vi "Teleop.vi"(10 "Match Info":T1={"Autonomous Elapsed Seconds"=0.0, "TeleOp Elapsed Seconds"=0.0, "Disabled Elapsed Seconds"=0.0, "Visited Autonomous"=FALSE, "Visited TeleOp"=FALSE, "Visited Disabled"=FALSE, "Autonomous Settings"={"Autonomous Style"=enum."Independent", "VI Refnum"=refnum}}, 11 "Call Context":T2) -> ()   [LabVIEW 2013]
doc: "This VI is called for each TeleOp packet received from the DS where the robot is not disabled. It is often used to read from the joysticks and update I/O or to update setpoints for timed control loops. It should complete and return within 20 milliseconds or it may miss DS packets."
uses:
  <vilib>/Rock Robotics/WPI/DriverStation/WPI_DriverStationDerivedRobotMode.ctl
  <vilib>/Rock Robotics/WPI/DriverStation/WPI_DriverStationMatch Info.ctl
  Robot Global Data.vi
  <vilib>/Rock Robotics/WPI/Joystick/WPI_JoystickGetSetRefNum.vi
panel:
  out "Button 12 Joy 4":bool
  out "Button 11 Joy 4":bool
  out "Button 10 Joy 4":bool
  out "Button 9 Joy 4":bool
  out "Button 8 Joy 4":bool
  out "Button 7 Joy 4":bool
  out "Button 6 Joy 4":bool
  out "Button 5 Joy 4":bool
  out "Button 4 Joy 4":bool
  out "Button 3 Joy 4":bool
  out "Button 2 Joy 4":bool
  out "Button 1 Joy 4":bool
  out "axis 4 Joy 4":dbl
  out "axis 3 (throttle) Joy 4":dbl
  out "axis 2 (y) Joy 4":dbl
  out "axis 1 (x) Joy 4":dbl
  out "Button 12 Joy 3":bool
  out "Button 11 Joy 3":bool
  out "Button 10 Joy 3":bool
  out "Button 9 Joy 3":bool
  out "Button 8 Joy 3":bool
  out "Button 7 Joy 3":bool
  out "Button 6 Joy 3":bool
  out "Button 5 Joy 3":bool
  out "Button 4 Joy 3":bool
  out "Button 3 Joy 3":bool
  out "Button 2 Joy 3":bool
  out "Button 1 Joy 3":bool
  out "axis 4 Joy 3":dbl
  out "axis 3 (throttle) Joy 3":dbl
  out "axis 2 (y) Joy 3":dbl
  out "axis 1 (x) Joy 3":dbl
  out "Button 12 Joy 2":bool
  out "Button 11 Joy 2":bool
  out "Button 10 Joy 2":bool
  out "Button 9 Joy 2":bool
  out "Button 8 Joy 2":bool
  out "Button 7 Joy 2":bool
  out "Button 6 Joy 2":bool
  out "Button 5 Joy 2":bool
  out "Button 4 Joy 2":bool
  out "Button 3 Joy 2":bool
  out "Button 2 Joy 2":bool
  out "Button 1 Joy 2":bool
  out "axis 4 Joy 2":dbl
  out "axis 3 (throttle) Joy 2":dbl
  out "axis 2 (y) Joy 2":dbl
  out "axis 1 (x) Joy 2":dbl
  out "Button 12 Joy 1":bool
  out "Button 11 Joy 1":bool
  out "Button 10 Joy 1":bool
  out "Button 9 Joy 1":bool
  out "Button 8 Joy 1":bool
  out "Button 7 Joy 1":bool
  out "Button 6 Joy 1":bool
  out "Button 5 Joy 1":bool
  out "Button 4 Joy 1":bool
  out "Button 3 Joy 1":bool
  out "Button 2 Joy 1":bool
  out "Button 1 Joy 1":bool
  out "axis 4 Joy":dbl
  out "axis 3 (throttle) Joy 1":dbl
  out "axis 2 (y) Joy 1":dbl
  out "axis 1 (x) Joy 1":dbl
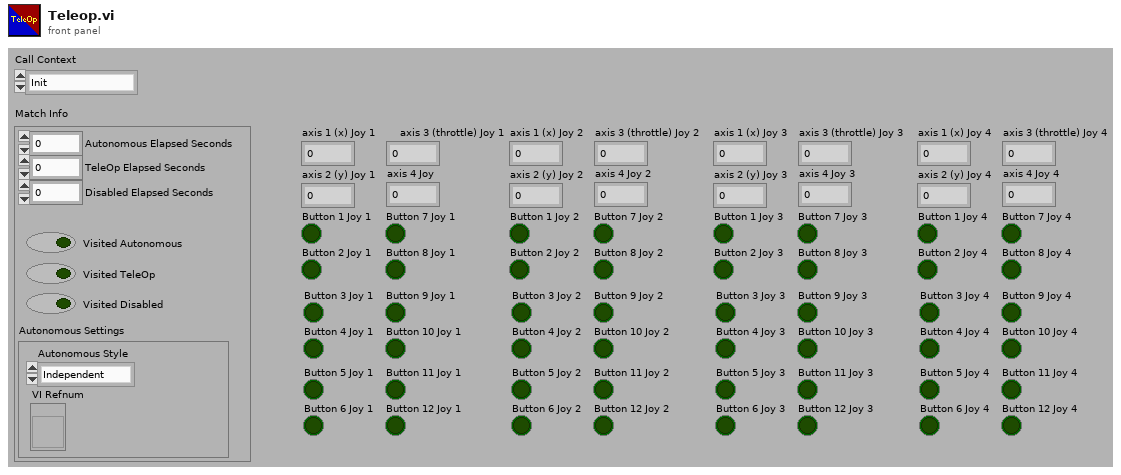
[diagram p1: front panel]
types:
  T1 = typedef "WPI_DriverStationMatch Info.ctl" = cluster{"Autonomous Elapsed Seconds":dbl, "TeleOp Elapsed Seconds":dbl, "Disabled Elapsed Seconds":dbl, "Visited Autonomous":bool, "Visited TeleOp":bool, "Visited Disabled":bool, "Autonomous Settings":cluster{"Autonomous Style":enum16{"Iterative", "Independent"}, "VI Refnum":refnum<vi>}}
  T2 = typedef "WPI_DriverStationDerivedRobotMode.ctl" = enum16{"Init", "Execute", "Stop"}
  T3 = typedef "WPI_JoystickDevRef.ctl" = cluster{"Device":T4}
  T4 = typedef "WPI_JoystickDeviceEnum.ctl" = enum16{"USB 1", "USB 2", "USB 3", "USB 4", "Kinect 1", "Kinect 2"}
  T5 = typedef "WPI_JoystickButtonState.ctl" = cluster{"Button 1":bool, "Button 2":bool, "Button 3":bool, "Button 4":bool, "Button 5":bool, "Button 6":bool, "Button 7":bool, "Button 8":bool, "Button 9":bool, "Button 10":bool, "Button 11":bool, "Button 12":bool}
  T6 = cluster{"axis 1 (x)":dbl, "axis 2 (y)":dbl, "axis 3 (throttle)":dbl, "axis 4":dbl, "axis 5":dbl, "axis 6":dbl}
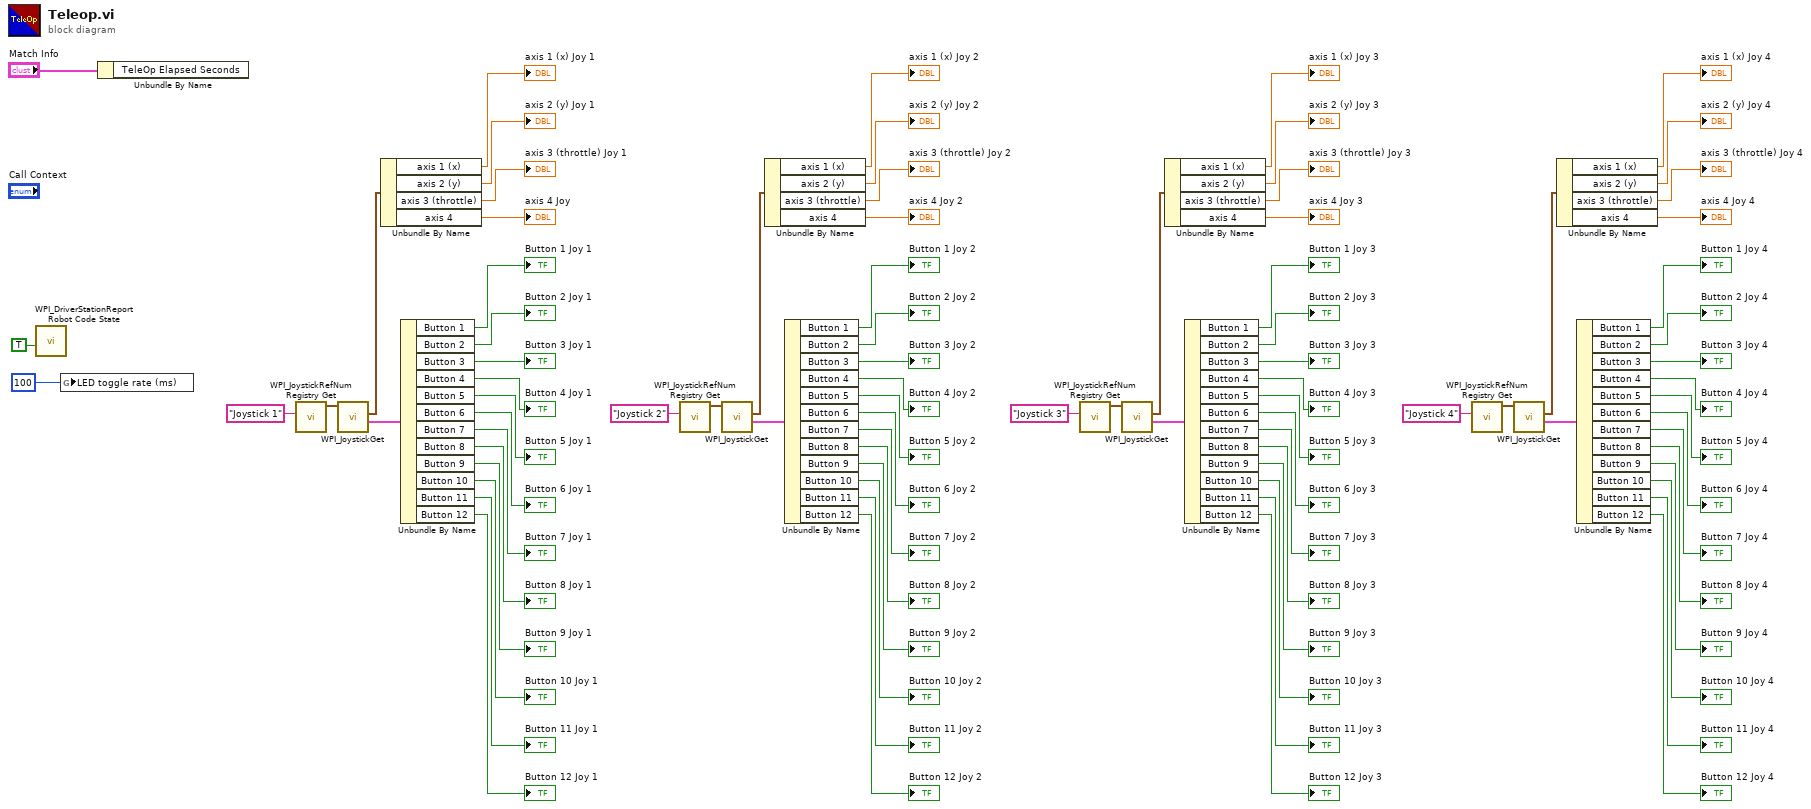
[diagram p0: block diagram]
diagram:
  n1 = call <vilib>:"WPI_DriverStationReport Robot Code State.vi"("TeleOp"=TRUE ("Autonomous")) -> ()  [unwired: 10 in, 1 out]
  n2 = global write "Robot Global Data.vi" "LED toggle rate (ms)"(u32 100 ("LED ms toggle rate")) -> ()
  n3 = Unbundle By Name("Match Info") -> ()  [unwired: 1 out]
  n4 = call <vilib>:"WPI_JoystickRefNum Registry Get.vi"("refnum name"="Joystick 1") -> ("JoystickDevRef"=w81:T3)  [unwired: 1 in, 9 out]
  n5 = call <vilib>:"WPI_JoystickGet.vi"("JoystickDevRef"=w81) -> ("Buttons"=w77:T5, "Axes"=w78:T6)  [unwired: 1 in, 4 out]
  n6 = Unbundle By Name(w78) -> ("axis 1 (x)"=→"axis 1 (x) Joy 1":dbl, "axis 2 (y)"=→"axis 2 (y) Joy 1":dbl, "axis 3 (throttle)"=→"axis 3 (throttle) Joy 1":dbl, "axis 4"=→"axis 4 Joy":dbl)
  n7 = Unbundle By Name(w77) -> ("Button 1"=→"Button 1 Joy 1":bool, "Button 2"=→"Button 2 Joy 1":bool, "Button 3"=→"Button 3 Joy 1":bool, "Button 4"=→"Button 4 Joy 1":bool, "Button 5"=→"Button 5 Joy 1":bool, "Button 6"=→"Button 6 Joy 1":bool, "Button 7"=→"Button 7 Joy 1":bool, "Button 8"=→"Button 8 Joy 1":bool, "Button 9"=→"Button 9 Joy 1":bool, "Button 10"=→"Button 10 Joy 1":bool, "Button 11"=→"Button 11 Joy 1":bool, "Button 12"=→"Button 12 Joy 1":bool)
  n8 = call <vilib>:"WPI_JoystickRefNum Registry Get.vi"("refnum name"="Joystick 2") -> ("JoystickDevRef"=w59:T3)  [unwired: 1 in, 9 out]
  n9 = call <vilib>:"WPI_JoystickGet.vi"("JoystickDevRef"=w59) -> ("Buttons"=w57:T5, "Axes"=w58:T6)  [unwired: 1 in, 4 out]
  n10 = Unbundle By Name(w58) -> ("axis 1 (x)"=→"axis 1 (x) Joy 2":dbl, "axis 2 (y)"=→"axis 2 (y) Joy 2":dbl, "axis 3 (throttle)"=→"axis 3 (throttle) Joy 2":dbl, "axis 4"=→"axis 4 Joy 2":dbl)
  n11 = Unbundle By Name(w57) -> ("Button 1"=→"Button 1 Joy 2":bool, "Button 2"=→"Button 2 Joy 2":bool, "Button 3"=→"Button 3 Joy 2":bool, "Button 4"=→"Button 4 Joy 2":bool, "Button 5"=→"Button 5 Joy 2":bool, "Button 6"=→"Button 6 Joy 2":bool, "Button 7"=→"Button 7 Joy 2":bool, "Button 8"=→"Button 8 Joy 2":bool, "Button 9"=→"Button 9 Joy 2":bool, "Button 10"=→"Button 10 Joy 2":bool, "Button 11"=→"Button 11 Joy 2":bool, "Button 12"=→"Button 12 Joy 2":bool)
  n12 = call <vilib>:"WPI_JoystickRefNum Registry Get.vi"("refnum name"="Joystick 3") -> ("JoystickDevRef"=w39:T3)  [unwired: 1 in, 9 out]
  n13 = call <vilib>:"WPI_JoystickGet.vi"("JoystickDevRef"=w39) -> ("Buttons"=w37:T5, "Axes"=w38:T6)  [unwired: 1 in, 4 out]
  n14 = Unbundle By Name(w38) -> ("axis 1 (x)"=→"axis 1 (x) Joy 3":dbl, "axis 2 (y)"=→"axis 2 (y) Joy 3":dbl, "axis 3 (throttle)"=→"axis 3 (throttle) Joy 3":dbl, "axis 4"=→"axis 4 Joy 3":dbl)
  n15 = Unbundle By Name(w37) -> ("Button 1"=→"Button 1 Joy 3":bool, "Button 2"=→"Button 2 Joy 3":bool, "Button 3"=→"Button 3 Joy 3":bool, "Button 4"=→"Button 4 Joy 3":bool, "Button 5"=→"Button 5 Joy 3":bool, "Button 6"=→"Button 6 Joy 3":bool, "Button 7"=→"Button 7 Joy 3":bool, "Button 8"=→"Button 8 Joy 3":bool, "Button 9"=→"Button 9 Joy 3":bool, "Button 10"=→"Button 10 Joy 3":bool, "Button 11"=→"Button 11 Joy 3":bool, "Button 12"=→"Button 12 Joy 3":bool)
  n16 = call <vilib>:"WPI_JoystickRefNum Registry Get.vi"("refnum name"="Joystick 4") -> ("JoystickDevRef"=w19:T3)  [unwired: 1 in, 9 out]
  n17 = call <vilib>:"WPI_JoystickGet.vi"("JoystickDevRef"=w19) -> ("Buttons"=w17:T5, "Axes"=w18:T6)  [unwired: 1 in, 4 out]
  n18 = Unbundle By Name(w18) -> ("axis 1 (x)"=→"axis 1 (x) Joy 4":dbl, "axis 2 (y)"=→"axis 2 (y) Joy 4":dbl, "axis 3 (throttle)"=→"axis 3 (throttle) Joy 4":dbl, "axis 4"=→"axis 4 Joy 4":dbl)
  n19 = Unbundle By Name(w17) -> ("Button 1"=→"Button 1 Joy 4":bool, "Button 2"=→"Button 2 Joy 4":bool, "Button 3"=→"Button 3 Joy 4":bool, "Button 4"=→"Button 4 Joy 4":bool, "Button 5"=→"Button 5 Joy 4":bool, "Button 6"=→"Button 6 Joy 4":bool, "Button 7"=→"Button 7 Joy 4":bool, "Button 8"=→"Button 8 Joy 4":bool, "Button 9"=→"Button 9 Joy 4":bool, "Button 10"=→"Button 10 Joy 4":bool, "Button 11"=→"Button 11 Joy 4":bool, "Button 12"=→"Button 12 Joy 4":bool)
